vi "Get Auto Range Value [ARV].vi"(8 "error in (no error)":errorcluster, 11 "CS++DMM in":refnum<class "CS++DMM.lvclass">) -> (0 "error out":errorcluster, 2 "actual range":dbl format="%^.2e", 3 "CS++DMM out":refnum<class "CS++DMM.lvclass">)   [LabVIEW 2013, in "CS++DMM.lvlib" / "CS++DMM.lvclass"]
doc: "This VI returns the actual range the DMM is currently using, even while it is auto-ranging.\n\nNote: \n\n(1) This VI is part of the IviDmmAutoRangeValue [ARV] extension group."
uses:
  CS++DMM.lvclass
  CSPP_Core/Classes/CS++ProcessVariables/ProcessVariable/PV.lvclass
  CSPP_Core/Classes/CS++ProcessVariables/ProcessVariable/PV.lvclass/PV.ctl
  CS++DMM.lvclass/CS++DMM.ctl
  CSPP_Core/Classes/CS++ProcessVariables/PVConnection/PVConnection.lvclass
  CSPP_Core/Classes/CS++ProcessVariables/ProcessVariable/Write Data.vi
  CSPP_Core/Classes/CS++ProcessVariables/ProcessVariable/Write Timestamp.vi
  CSPP_Core/Classes/CS++ProcessVariables/ProcessVariable/Write Quality.vi
  CSPP_Core/Classes/CS++ProcessVariables/ProcessVariable/Write status.vi
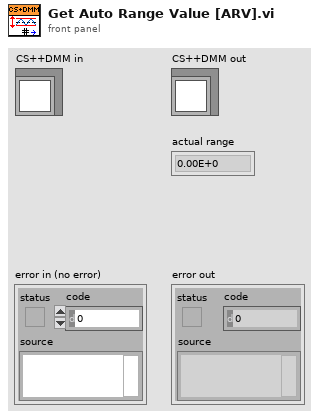
[diagram p1: front panel]
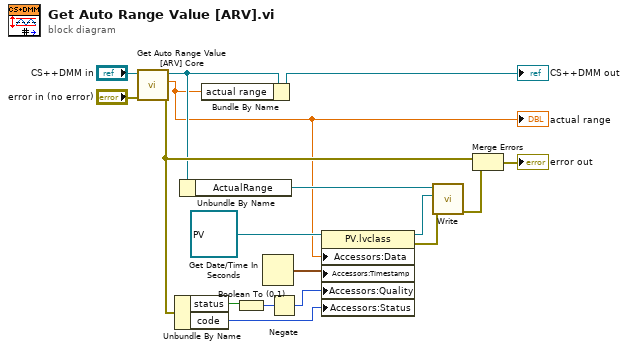
[diagram p0: block diagram]
diagram:
  n1 = call-dynamic "Get Auto Range Value [ARV] Core.vi"("error in (no error)"="error in (no error)", "CS++DMM in"="CS++DMM in") -> ("error out"=w6:errorcluster, "actual range"=w1:dbl, "CS++DMM out"=w3:refnum<class "CS++DMM.lvclass">)  [unwired: 7 in]
  "actual range" <- w1
  n2 = Unbundle By Name(w6) -> ("status"=w15:bool, "code"=w12:i32)
  n3 = Unbundle By Name(w3) -> ("ActualRange"=w17:refnum<class "PVConnection.lvclass">)
  n4 = Bundle By Name(cluster=w3, "actual range"=w1) -> (→"CS++DMM out":refnum<class "CS++DMM.lvclass">)
  n5 = Boolean To (0,1)(Boolean=w15) -> (0, 1=w14:i16)
  n6 = Get Date/Time In Seconds() -> (seconds since 1Jan1904=w11:timestamp)
  n7 = Negate(x=w14) -> (-x=w13:i16)
  n8 = property class="PV.lvclass"(reference=refnum<class "PV.lvclass"> refnum ("CS++ProcessVariables.lvlib:PV.lvclass"), "Accessors:Data"=w1, "Accessors:Timestamp"=w11, "Accessors:Quality"=w13, "Accessors:Status"=w12) -> (reference out=w10:refnum<class "PV.lvclass">, error out=w9:errorcluster)  [unwired: 1 in]
  n9 = call-dynamic "Write.vi"("error in (no error)"=w9, "PV"=w10, "PVConnection in"=w17) -> ("error out"=w4:errorcluster)  [unwired: 7 in, 1 out]
  n10 = Merge Errors(w6, w4) -> (→"error out":errorcluster)
